vi "Create msTick LogFile.vi"(8 "error in (no error)":errorcluster, 11 "DbgTimers in":refnum<class "DbgTimers.lvclass">) -> (0 "error out":errorcluster, 2 "LogFile path":path, 3 "DbgTimers out":refnum<class "DbgTimers.lvclass">)   [LabVIEW 2017, in "DbgTimers.lvclass"]
doc: "Developed by Kevin Thompson\nkevin@thompsonengineering.net\n\nCopyright 2018-2020\nThompson Engineering, LLC"
uses:
  DbgTimers.lvclass
  DbgTimers.lvclass/DbgTimers.ctl
  Accessors/Get ObjData.vi
  Accessors/Set LogFile_msTickTimer.vi
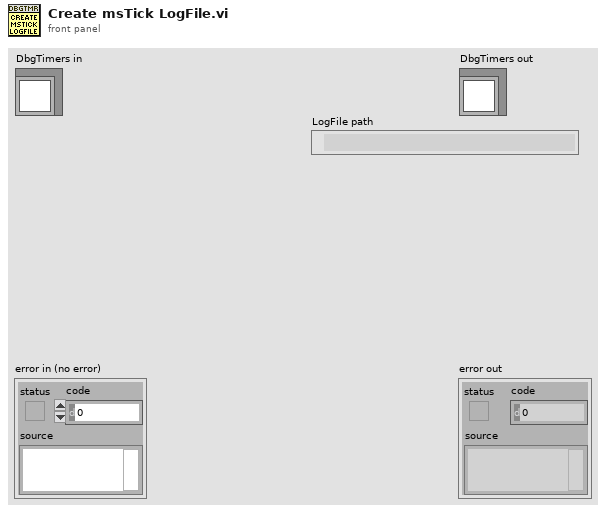
[diagram p1: front panel]
types:
  T1 = typedef "DbgTimers.lvclass/ObjData--cluster.ctl" = cluster{"Settings":T2, "ReadData-placeholder":T3, "Timers":T4, "Enable msTick Logging":bool, "LogFile_msTickTimer":path}
  T2 = typedef "DbgTimers.lvclass/Settings--cluster.ctl" = cluster{"Simulation":bool, "DbgTimer LogFolder":path}
  T3 = typedef "DbgTimers.lvclass/Read Data--cluster.ctl" = cluster{"Data":dbl}
  T4 = typedef "DbgTimers.lvclass/Timers--cluster.ctl" = cluster{"ms tick timers":T5[]}
  T5 = typedef "DbgTimers.lvclass/Millisecond Tick Timer--cluster.ctl" = cluster{"startTick":u32, "currentTick":u32, "elapsedTicks":u32, "totalElapsedTicks":u32}
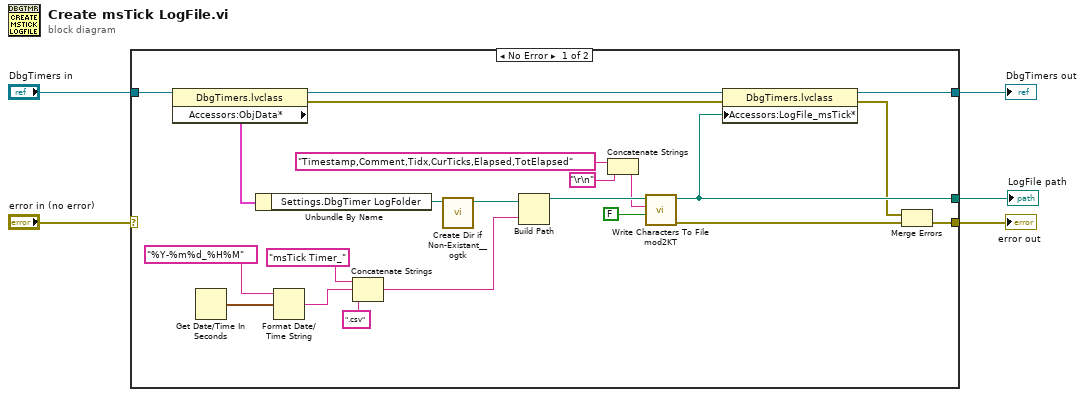
[diagram p0: block diagram]
diagram:
  n1 = case shown="No Error" "error in (no error)" {
    selector: "error in (no error)" -> [_ w29]
    tunnel: [w13 w29] -> w4
    tunnel: [w12 w28] -> w2
    tunnel: "DbgTimers in" -> [w27 w28]
    tunnel: [w11 _] -> w1
    frame No Error {
      n2 = property class="DbgTimers.lvclass"(reference=w27) -> (reference out=w26:refnum<class "DbgTimers.lvclass">, error out=w10:errorcluster, "Accessors:ObjData*"=w25:T1)  [unwired: 1 in]
      n3 = Get Date/Time In Seconds() -> (seconds since 1Jan1904=w18:timestamp)
      n4 = Unbundle By Name(w25) -> ("Settings.DbgTimer LogFolder"=w24:path)
      n5 = Format Date/Time String(time format string (%c)="%Y-%m%d_%H%M", seconds (now)=w18) -> (date/time string=w21:string)  [unwired: 1 in]
      n6 = Concatenate Strings("msTick Timer_" ("string"), w21, ".csv" ("string")) -> (w17:string)
      n7 = call <userlib>:"Create Dir if Non-Existant__ogtk.vi"("Directory Path"=w24) -> ("dup Directory Path"=w23:path)  [unwired: 8 in, 2 out]
      n8 = Build Path(base path=w23, name or relative path=w17) -> (appended path=w16:path)
      n9 = Concatenate Strings("Timestamp,Comment,Tidx,CurTicks,Elapsed,TotElapsed", "\r\n") -> (w6:string)
      n10 = call <vilib>:"Write Characters To File mod2KT.vi"("advisory dialog? (display:T)"=FALSE, "character string"=w6, "file path (dialog if empty)"=w16) -> ("error out"=w14:errorcluster, "new file path (Not A Path if cancelled)"=w11:path)  [unwired: 3 in]
      n11 = property class="DbgTimers.lvclass"(reference=w26, error in=w10, "Accessors:LogFile_msTick*"=w11) -> (reference out=w12:refnum<class "DbgTimers.lvclass">, error out=w9:errorcluster)
      n12 = Merge Errors(w9, w14) -> (w13:errorcluster)
    }
    frame Error {
    }
  }
  "error out" <- w4
  "DbgTimers out" <- w2
  "LogFile path" <- w1
